vi "Get Follow Wall Target Position.vi"(8 "Wall left?":bool, 9 "Target Distance":dbl=220.0) -> (2 "Target Y (Relative)":dbl, 3 "Target X (Relative)":dbl)   [LabVIEW 2017]
uses:
  Globals/Pose.vi
panel:
  out "Wall distance":dbl=213.6
  out "Wall error":dbl=6.400000000000006
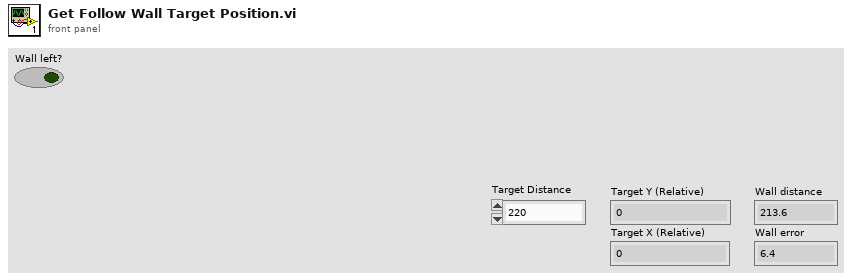
[diagram p1: front panel]
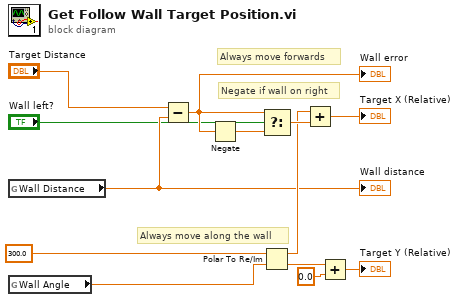
[diagram p0: block diagram]
diagram:
  # "Always move along the wall"
  # "Negate if wall on right"
  # "Always move forwards"
  n1 = global read "Pose.vi" "Wall Distance"() -> (w6:dbl)
  "Wall distance" <- w6
  n2 = global read "Pose.vi" "Wall Angle"() -> (w12:dbl)
  n3 = Subtract(x="Target Distance", y=w6) -> (x-y=w9:dbl)
  "Wall error" <- w9
  n4 = Negate(x=w9) -> (-x=w8:dbl)
  n5 = Select(t=w9, s="Wall left?", f=w8) -> (s? t:f=w13:dbl)
  n6 = Polar To Re/Im(2:w12, 3:300.0 ("r")) -> (0:w10:dbl, 1:w11:dbl)
  n7 = Add(x=w11, y=w13) -> (x+y=→"Target X (Relative)":dbl)
  n8 = Add(x=w10, y=0.0) -> (x+y=→"Target Y (Relative)":dbl)
